vi "Edit and Save Key Variable.vi"() -> ()   [LabVIEW 2015]
uses:
  <vilib>/Utility/config.llb/Write Key (String).vi
  <vilib>/Utility/config.llb/NI_LVConfig.lvlib
panel:
  in  "Save":bool
  in  "Preferences":string[][](array[string])
  in  "Cancel":bool
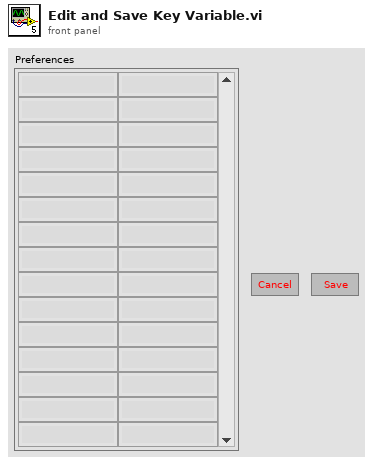
[diagram p1: front panel]
types:
  T1 = typedef "NI_LVConfig.lvlib/Config Data RefNum.ctl" = refnum<k1>
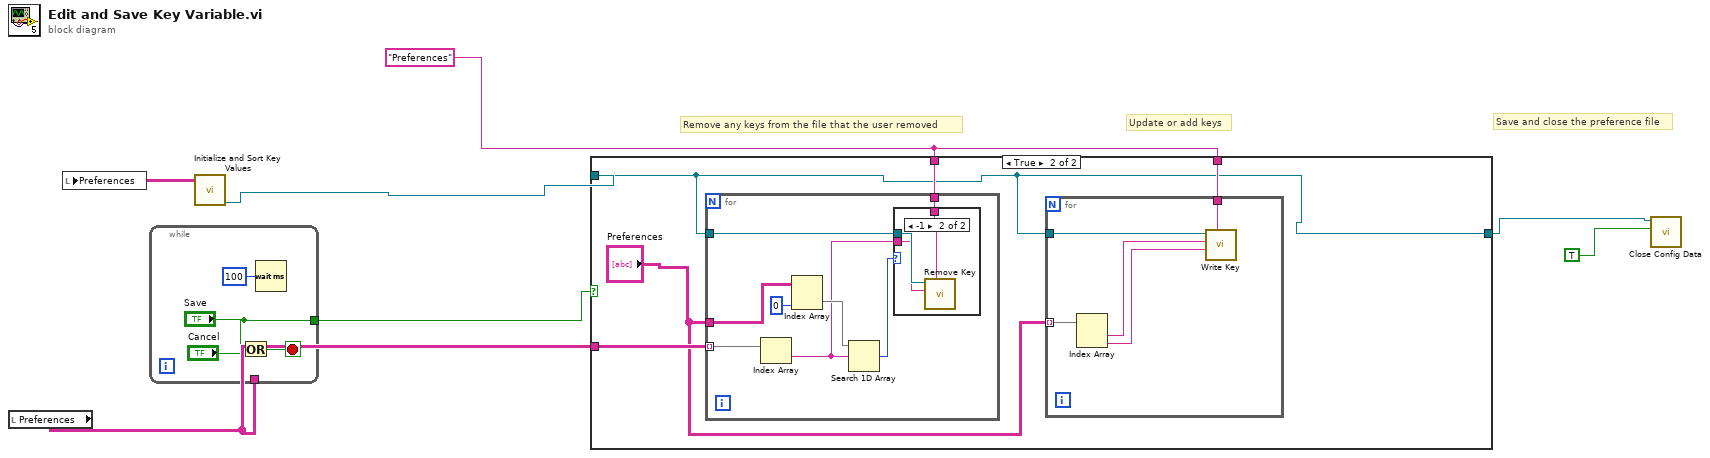
[diagram p0: block diagram]
diagram:
  w2 = "Preferences" ("section")
  # "Save and close the preference file"
  # "Update or add keys"
  # "Remove any keys from the file that the user removed"
  n1 = local read "Preferences"() -> (w4:string[][])
  n2 = while {
    tunnel: ["Save"] -> w3
    tunnel: w4 -> [_]
    stop <- w10 stop-if-true
    n3 = Or(x="Save", y="Cancel") -> (x .or. y?=w10:bool)
    n4 = Wait (ms)(milliseconds to wait=u32 100) -> ()  [unwired: 1 out]
  }
  n5 = call "Initialize and Sort Key Values.vi"() -> ("refnum"=w1:T1, "Preferences"=w7:string[][])  [unwired: 10 in]
  n6 = local write "Preferences"(w7) -> ()
  n7 = case shown="True" w3 {
    tunnel: w1 -> [w12 w13]
    tunnel: w4 -> [_ w17]
    tunnel: w2 -> [_ w16]
    tunnel: [w12 w13] -> w6
    tunnel: w2 -> [_ w15]
    frame False {
    }
    frame True {
      n8 = for {
        tunnel: w13 -> [w27]
        tunnel: w17 -> [w30] mode=indexing
        tunnel: w16 -> [w26]
        tunnel: "Preferences" -> [w23]
        n9 = Index Array(array=w30) -> (element=w25:string)  [unwired: 1 in]
        n10 = Index Array(array=w23, index (col)=0 ("disabled index (col)")) -> (element=w28:string[])  [unwired: 1 in]
        n11 = Search 1D Array(1D array=w28, element=w25) -> (index of element=w24:i32)  [unwired: 1 in]
        n12 = case shown="-1" w24 {
          tunnel: w27 -> [_ w33]
          tunnel: w26 -> [_ w32]
          tunnel: w25 -> [_ w31]
          frame 0, Default {
          }
          frame -1 {
            n13 = call <vilib>:"Remove Key.vi"("section"=w32, "key"=w31, "refnum"=w33) -> ()  [unwired: 6 in, 3 out]
          }
        }
      }
      n14 = for {
        tunnel: "Preferences" -> [w22] mode=indexing
        tunnel: w13 -> [w18]
        tunnel: w15 -> [w21]
        n15 = Index Array(array=w22) -> (element #1=w20:string, element #2=w19:string)  [unwired: 2 in]
        n16 = call-poly <vilib>:"Write Key.vi"("section"=w21, "value"=w19, "key"=w20, "refnum"=w18) -> ()  [unwired: 5 in, 3 out]
      }
    }
  }
  n17 = call <vilib>:"Close Config Data.vi"("write file if changed (T)"=TRUE, "refnum"=w6) -> ()  [unwired: 8 in, 2 out]
